vi "Usando VIs.vi"   [LabVIEW 2020]
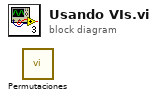
[diagram p0: block diagram]
diagram:
  n1 = call "Permutaciones.vi"() -> ()  [unwired: 11 in, 1 out]
